vi "SDCP BTR Start.vi"(3 "error in (no error)":errorcluster, 4 "Number of transfers":u16, 5 "Parameter IDs":u8[](array[numeric])) -> (0 "error out":errorcluster, 1 "No timeout":bool, 2 "out":T1)   [LabVIEW 2020]
uses:
  Typedefs/SDCP BTR Params.ctl
  <vilib>/Instr/_visa.llb/VISA Flush IO Buffer Mask.ctl
  Typedefs/SDCP - Serial Port Control - Commands.ctl
panel:
  in  "COM Port":refnum<visa-resource-name>
  in  "Baud rate":u32=9600
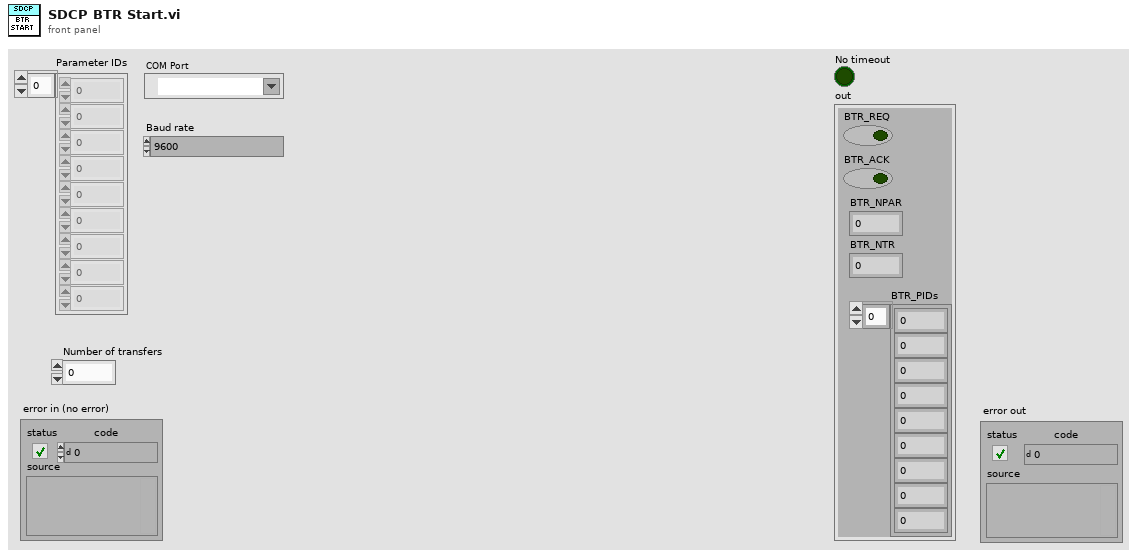
[diagram p1: front panel]
types:
  T1 = typedef "SDCP BTR Params.ctl" = cluster{"BTR_REQ":bool, "BTR_ACK":bool, "BTR_NPAR":i32, "BTR_NTR":i32, "BTR_PIDs":u8[]}
  T2 = typedef "SDCP - Serial Port Control - Commands.ctl" = enum16{"Open", "Read", "Write", "Get instance", "Close"}
  T3 = typedef "VISA Flush IO Buffer Mask.ctl" = u16
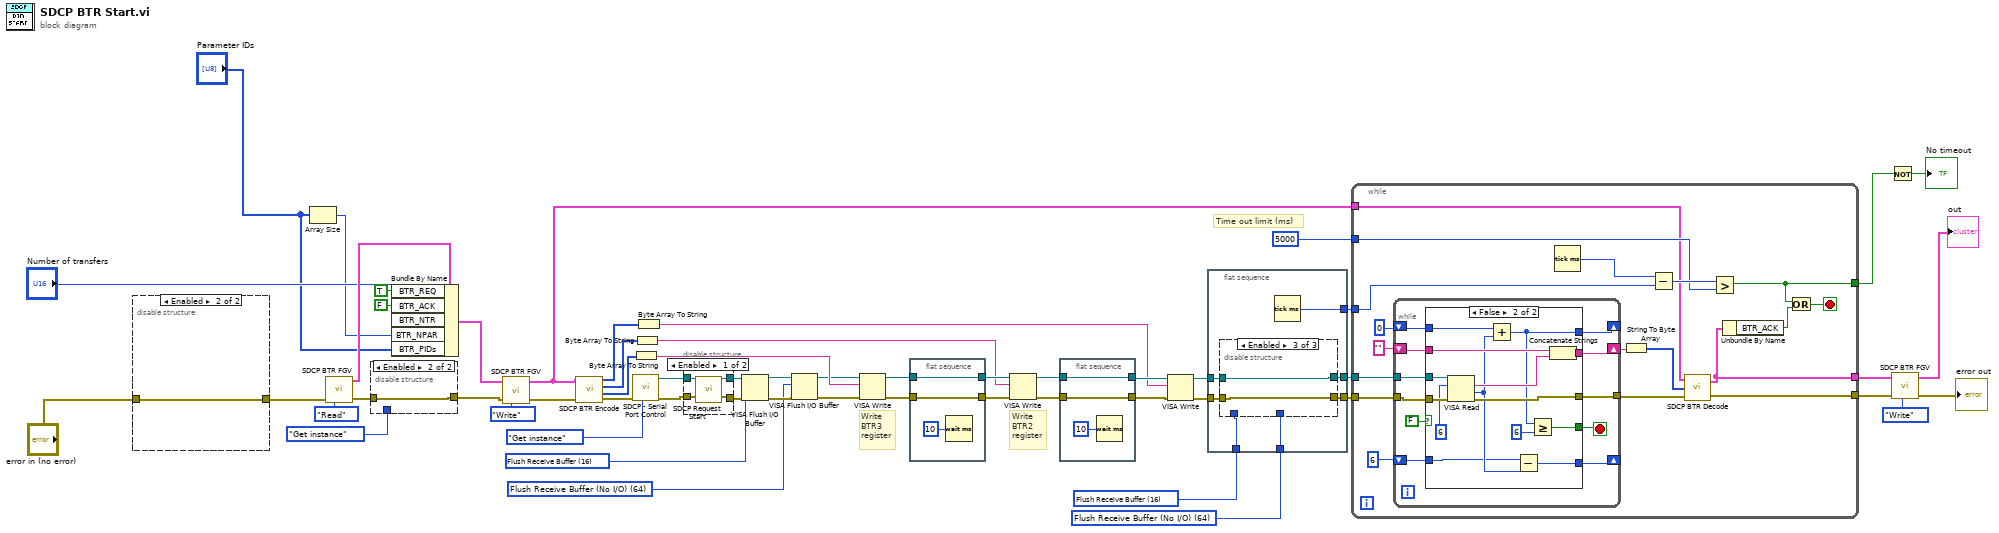
[diagram p0: block diagram]
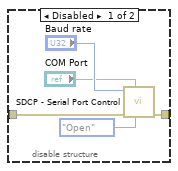
[diagram p2: hidden frame]
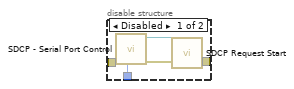
[diagram p3: hidden frame]
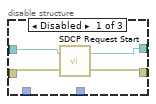
[diagram p4: hidden frame]
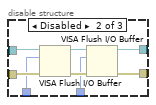
[diagram p5: hidden frame]
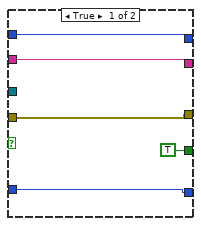
[diagram p7: hidden frame]
diagram:
  w27 = T3 64 items=["Flush Receive Buffer"=16, "Write Transmit Buffer to Device"=32, "Flush Receive Buffer (No I/O)"=64, "Flush Transmit Buffer"=128] ("Mask")
  w28 = T3 16 items=["Flush Receive Buffer"=16, "Write Transmit Buffer to Device"=32, "Flush Receive Buffer (No I/O)"=64, "Flush Transmit Buffer"=128] ("Mask")
  w45 = T3 64 items=["Flush Receive Buffer"=16, "Write Transmit Buffer to Device"=32, "Flush Receive Buffer (No I/O)"=64, "Flush Transmit Buffer"=128] ("Mask")
  w48 = T3 16 items=["Flush Receive Buffer"=16, "Write Transmit Buffer to Device"=32, "Flush Receive Buffer (No I/O)"=64, "Flush Transmit Buffer"=128] ("Mask")
  # "Time out limit (ms)"
  # "Write\nBTR2\nregister"
  # "Write\nBTR3\nregister"
  n1 = disable-structure shown="Enabled" {
    disable-tunnel: [w62 w63] -> w2
    disable-tunnel: "error in (no error)" -> [w61 w63]
    frame Disabled {
      n2 = call "SDCP - Serial Port Control.vi"("Command"=SDCP_-_Serial_Port_Control_-_Commands."Open", "VISA resource name"="COM Port", "error in (no error)"=w61, "Baud rate"="Baud rate") -> ("error out"=w62:errorcluster)  [unwired: 4 in, 3 out]
    }
    frame Enabled {
    }
  }
  n3 = Array Size(array="Parameter IDs") -> (size(s)=w52:i32)
  n4 = call "SDCP BTR FGV.vi"("error in (no error)"=w2, "Command"=enum16{"Read", "Write"}."Read") -> ("error out"=w5:errorcluster, "out"=w56:T1)  [unwired: 2 in]
  n5 = disable-structure shown="Enabled" {
    disable-tunnel: w5 -> [w68 w69]
    disable-tunnel: SDCP_-_Serial_Port_Control_-_Commands."Get instance" ("Command") -> [w67 _]
    disable-tunnel: [w64 w69] -> w3
    frame Disabled {
      n6 = call "SDCP - Serial Port Control.vi"("Command"=w67, "error in (no error)"=w68) -> ("error out"=w66:errorcluster, "VISA out"=w65:refnum<visa-resource-name>)  [unwired: 6 in, 2 out]
      n7 = call "SDCP Request Start.vi"("error in (no error)"=w66, "COM Port"=w65) -> ("error out"=w64:errorcluster)  [unwired: 1 out]
    }
    frame Enabled {
    }
  }
  n8 = Bundle By Name(cluster=w56, "BTR_REQ"=TRUE, "BTR_ACK"=FALSE, "BTR_NTR"="Number of transfers", "BTR_NPAR"=w52, "BTR_PIDs"="Parameter IDs") -> (w20:T1)
  n9 = call "SDCP BTR FGV.vi"("error in (no error)"=w3, "Command"=enum16{"Read", "Write"}."Write", "in"=w20) -> ("error out"=w18:errorcluster, "out"=w17:T1)  [unwired: 1 in]
  n10 = call "SDCP BTR Encode.vi"("error in (no error)"=w18, "in"=w17) -> ("error out"=w50:errorcluster, "BTR3 encoded"=w43:u8[], "BTR2 encoded"=w38:u8[], "BTR1 encoded"=w37:u8[])  [unwired: 2 in]
  n11 = call "SDCP - Serial Port Control.vi"("Command"=SDCP_-_Serial_Port_Control_-_Commands."Get instance", "error in (no error)"=w50) -> ("error out"=w9:errorcluster, "VISA out"=w8:refnum<visa-resource-name>)  [unwired: 6 in, 2 out]
  n12 = Byte Array To String(unsigned byte array=w43) -> (string=w42:string)
  n13 = Byte Array To String(unsigned byte array=w38) -> (string=w32:string)
  n14 = Byte Array To String(unsigned byte array=w37) -> (string=w29:string)
  n15 = disable-structure shown="Enabled" {
    disable-tunnel: w9 -> [w73 w74]
    disable-tunnel: w8 -> [w72 w75]
    disable-tunnel: [w71 w74] -> w7
    disable-tunnel: [w70 w75] -> w6
    frame Enabled {
      n16 = call "SDCP Request Start.vi"("error in (no error)"=w73, "COM Port"=w72) -> ("error out"=w71:errorcluster, "COM Port Out"=w70:refnum<visa-resource-name>)
    }
    frame Disabled {
    }
  }
  n17 = VISA Flush I/O Buffer(VISA resource name=w6, mask (16)=w48, error in (no error)=w7) -> (VISA resource name out=w46:refnum<visa-resource-name>, error out=w47:errorcluster)
  n18 = VISA Flush I/O Buffer(VISA resource name=w46, mask (16)=w45, error in (no error)=w47) -> (VISA resource name out=w41:refnum<visa-resource-name>, error out=w44:errorcluster)
  n19 = VISA Write(VISA resource name=w41, write buffer=w42, error in (no error)=w44) -> (VISA resource name out=w39:refnum<visa-resource-name>, error out=w40:errorcluster)  [unwired: 1 out]
  n20 = flat-sequence {
    tunnel: w40 -> [w77]
    tunnel: [w77] -> w34
    tunnel: w39 -> [w76]
    tunnel: [w76] -> w33
    frame #0 {
      n21 = Wait (ms)(milliseconds to wait=u32 10) -> ()  [unwired: 1 out]
    }
  }
  n22 = VISA Write(VISA resource name=w33, write buffer=w32, error in (no error)=w34) -> (VISA resource name out=w35:refnum<visa-resource-name>, error out=w36:errorcluster)  [unwired: 1 out]
  n23 = flat-sequence {
    tunnel: w36 -> [w80]
    tunnel: [w80] -> w31
    tunnel: w35 -> [w79]
    tunnel: [w79] -> w30
    frame #0 {
      n24 = Wait (ms)(milliseconds to wait=u32 10) -> ()  [unwired: 1 out]
    }
  }
  n25 = VISA Write(VISA resource name=w30, write buffer=w29, error in (no error)=w31) -> (VISA resource name out=w25:refnum<visa-resource-name>, error out=w26:errorcluster)  [unwired: 1 out]
  n26 = flat-sequence {
    tunnel: w28 -> [w88]
    tunnel: w27 -> [w87]
    tunnel: w26 -> [w86]
    tunnel: w25 -> [w85]
    tunnel: [w84] -> w24
    tunnel: [w83] -> w23
    tunnel: [w82] -> w21
    frame #0 {
      n27 = disable-structure shown="Enabled" {
        disable-tunnel: w88 -> [_ w98 _]
        disable-tunnel: w87 -> [_ w93 _]
        disable-tunnel: w86 -> [w91 w99 w101]
        disable-tunnel: w85 -> [w92 w100 w102]
        disable-tunnel: [w89 w94 w101] -> w84
        disable-tunnel: [w90 w95 w102] -> w83
        frame Disabled {
          n28 = call "SDCP Request Start.vi"("error in (no error)"=w91, "COM Port"=w92) -> ("error out"=w89:errorcluster, "COM Port Out"=w90:refnum<visa-resource-name>)
        }
        frame Disabled {
          n29 = VISA Flush I/O Buffer(VISA resource name=w100, mask (16)=w98, error in (no error)=w99) -> (VISA resource name out=w97:refnum<visa-resource-name>, error out=w96:errorcluster)
          n30 = VISA Flush I/O Buffer(VISA resource name=w97, mask (16)=w93, error in (no error)=w96) -> (VISA resource name out=w95:refnum<visa-resource-name>, error out=w94:errorcluster)
        }
        frame Enabled {
        }
      }
      n31 = Tick Count (ms)() -> (millisecond timer value=w82:u32)
    }
  }
  n32 = while {
    tunnel: w24 -> [w120]
    tunnel: w23 -> [w117]
    tunnel: 5000 -> [w113]
    tunnel: w21 -> [w116]
    tunnel: w17 -> [w110]
    tunnel: [w107] -> w16
    tunnel: [w106] -> w15
    tunnel: [w104] -> w11
    stop <- w109 stop-if-true
    n33 = while {
      tunnel: w120 -> [w131]
      shift-right: [w128] -> w112
      shift-left: "" -> [w129]
      shift-right: [w124] -> _
      shift-left: 0 -> [w126]
      tunnel: w117 -> [w130]
      tunnel: [w127] -> w111
      shift-right: [w123] -> _
      shift-left: u32 6 ("byte count") -> [w122]
      stop <- w125 stop-if-true
      n34 = case shown="False" FALSE {
        tunnel: w131 -> [w134 w150]
        tunnel: w130 -> [_ w149]
        tunnel: w129 -> [w135 w148]
        tunnel: [w135 w146] -> w128
        tunnel: [w134 w145] -> w127
        tunnel: w126 -> [w136 w144]
        tunnel: [TRUE w143] -> w125
        tunnel: [w136 w142] -> w124
        tunnel: [w133 w140] -> w123
        tunnel: w122 -> [w133 w139]
        frame True {
        }
        frame False {
          n35 = VISA Read(VISA resource name=w149, byte count=u32 6, error in (no error)=w150) -> (read buffer=w147:string, return count=w141:u32, error out=w145:errorcluster)  [unwired: 1 out]
          n36 = Add(x=w144, y=w141) -> (x+y=w142:u32)
          n37 = Subtract(x=w139, y=w141) -> (x-y=w140:u32)
          n38 = Greater Or Equal?(x=w142, y=u32 6 ("byte count")) -> (x >= y?=w143:bool)
          n39 = Concatenate Strings(w148, w147) -> (w146:string)
        }
      }
    }
    n40 = Tick Count (ms)() -> (millisecond timer value=w115:u32)
    n41 = String To Byte Array(string=w112) -> (unsigned byte array=w103:u8[])
    n42 = Subtract(x=w115, y=w116) -> (x-y=w114:u32)
    n43 = call "SDCP BTR Decode.vi"("error in (no error)"=w111, "Frame"=w103, "in"=w110) -> ("error out"=w107:errorcluster, "out"=w106:T1)
    n44 = Greater?(x=w114, y=w113) -> (0:w104:bool)
    n45 = Unbundle By Name(w106) -> ("BTR_ACK"=w108:bool)
    n46 = Or(x=w104, y=w108) -> (x .or. y?=w109:bool)
  }
  n47 = Not(x=w11) -> (.not. x?=→"No timeout":bool)
  n48 = call "SDCP BTR FGV.vi"("error in (no error)"=w16, "Command"=enum16{"Read", "Write"}."Write", "in"=w15) -> ("error out"=→"error out":errorcluster, "out"=→"out":T1)  [unwired: 1 in]
